vi "生成word报表.vi"(0 "Array输入":refnum<vi>, 1 "产品序号":string, 2 "标注图":T1(plugin-control), 3 "Array输入 2":refnum<vi>, 4 "测试人":string, 5 "部位":string, 6 "ROI左上角X":i32, 7 "ROI左上角Y":i32, 8 "反射图":T1(plugin-control) caption="Original Image", 9 "框号":dbl format="%#_13g") -> (14 "报告生成路径":path)   [LabVIEW 2018]
uses:
  <vilib>/Utility/NIReport.llb/Report Type.ctl
  <vilib>/Utility/NIReport.llb/Append Report Text (str wrap).vi
  <vilib>/addons/_office/word.llb/Word Edit Cell ([dbl]).vi
  <vilib>/addons/_office/word.llb/Word Edit Cell (str).vi
  <vilib>/Utility/NIReport.llb/Append Report Text (num wrap).vi
  <vilib>/Utility/NIReport.llb/NI_report.lvclass
  <vilib>/addons/_office/NI_ReportGenerationToolkit.lvlib
  <vilib>/Utility/NIReport.llb/Word/NI_Word.lvclass
  <vilib>/Utility/NIReport.llb/NI_ReportGenerationCore.lvlib
  <vilib>/addons/_office/word.llb/Word Edit Cell ([str]).vi
panel:
  out "绝对位置Y2":dbl[](array[numeric])
  out "绝对位置X2":dbl[](array[numeric])
  out "绝对位置Y":dbl[](array[numeric])
  out "绝对位置X":dbl[](array[numeric])
  out "分层累计缺陷占比":dbl
  out "分层Z值":dbl[](array[numeric])
  out "缺陷个数 2":i32
  out "分层数据":dbl[][](array[numeric])
  out "弥散累计缺陷占比":dbl
  out "弥散数据":dbl[][](array[numeric])
  out "弥散Z值":dbl[](array[numeric])
  out "缺陷个数":i32
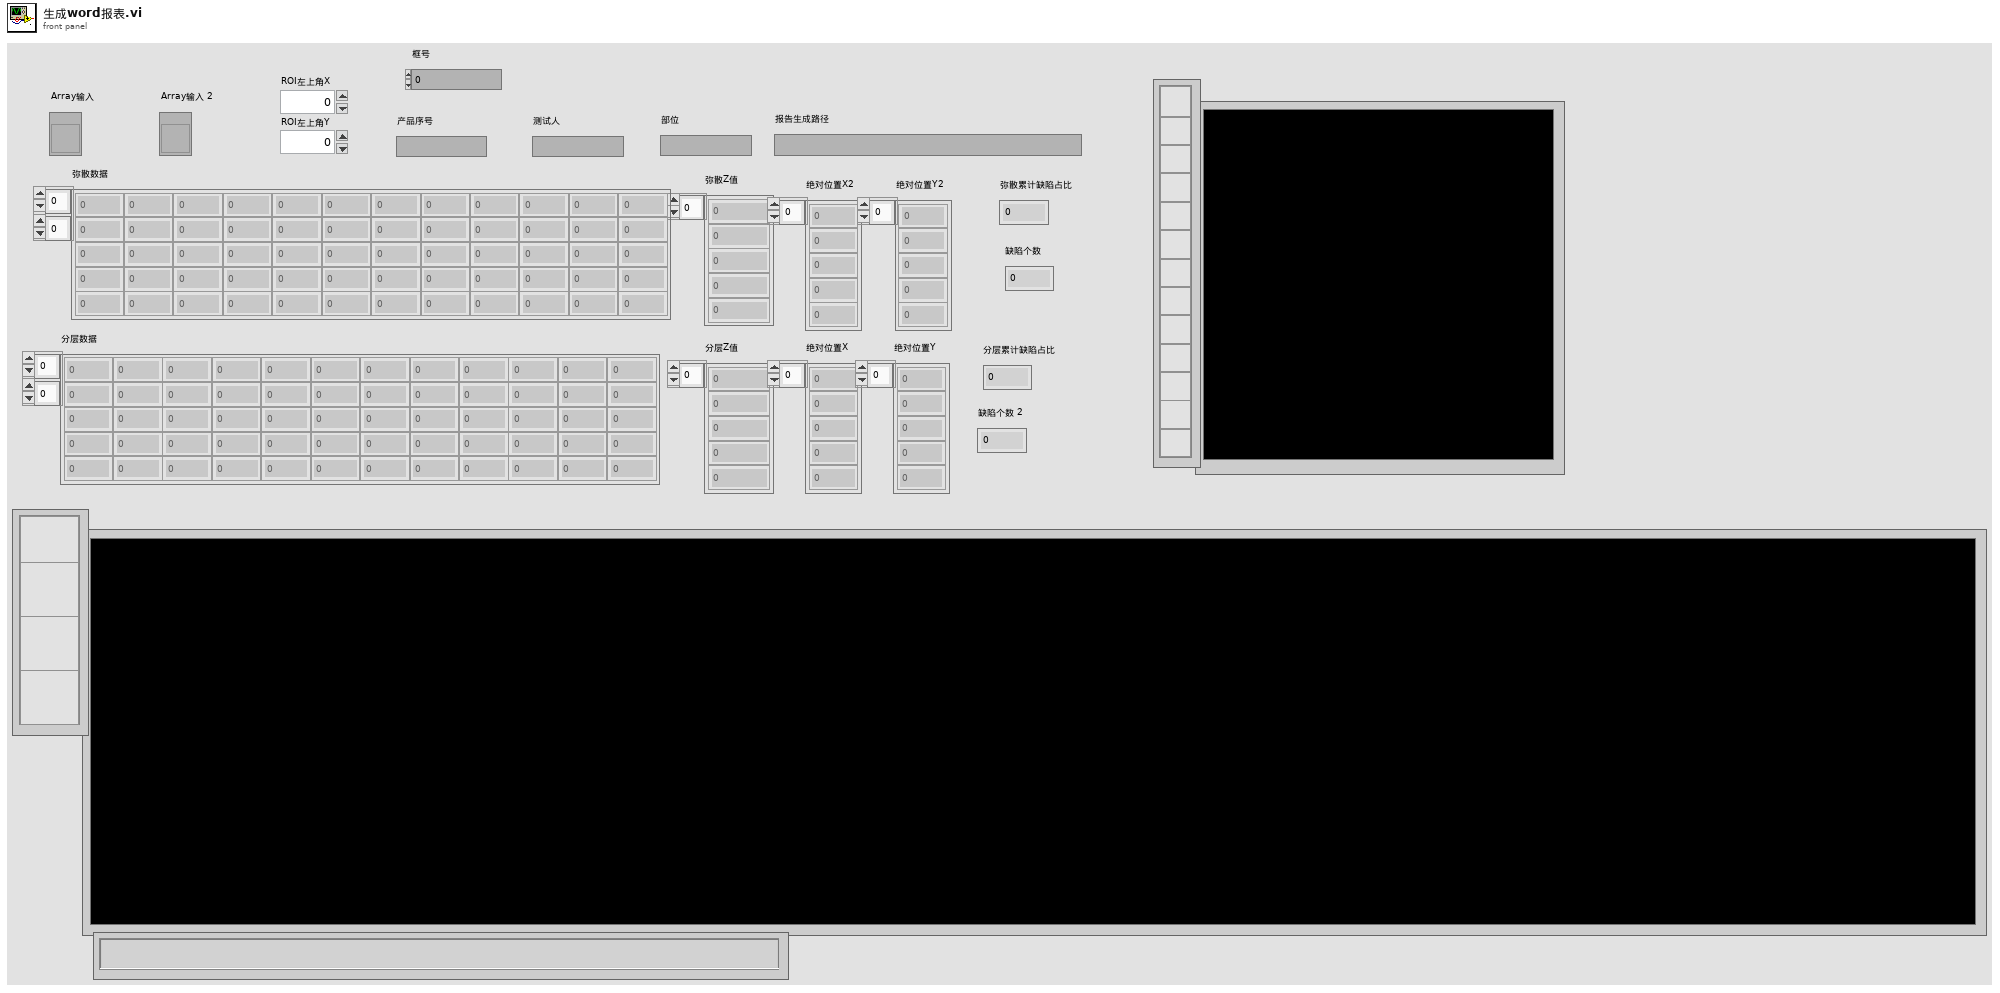
[diagram p1: front panel]
types:
  T1 = typedef "IMAQ Image.ctl" = refnum<image>
  T2 = cluster{"position (Excel)":cluster{"row":i32, "column":i32}, "name (Excel)":string, "bookmark (Word)":string}
  T3 = typedef "NI_ReportGenerationCore.lvlib/Report Type.ctl" = enum16{"HTML", "Word", "Excel"}
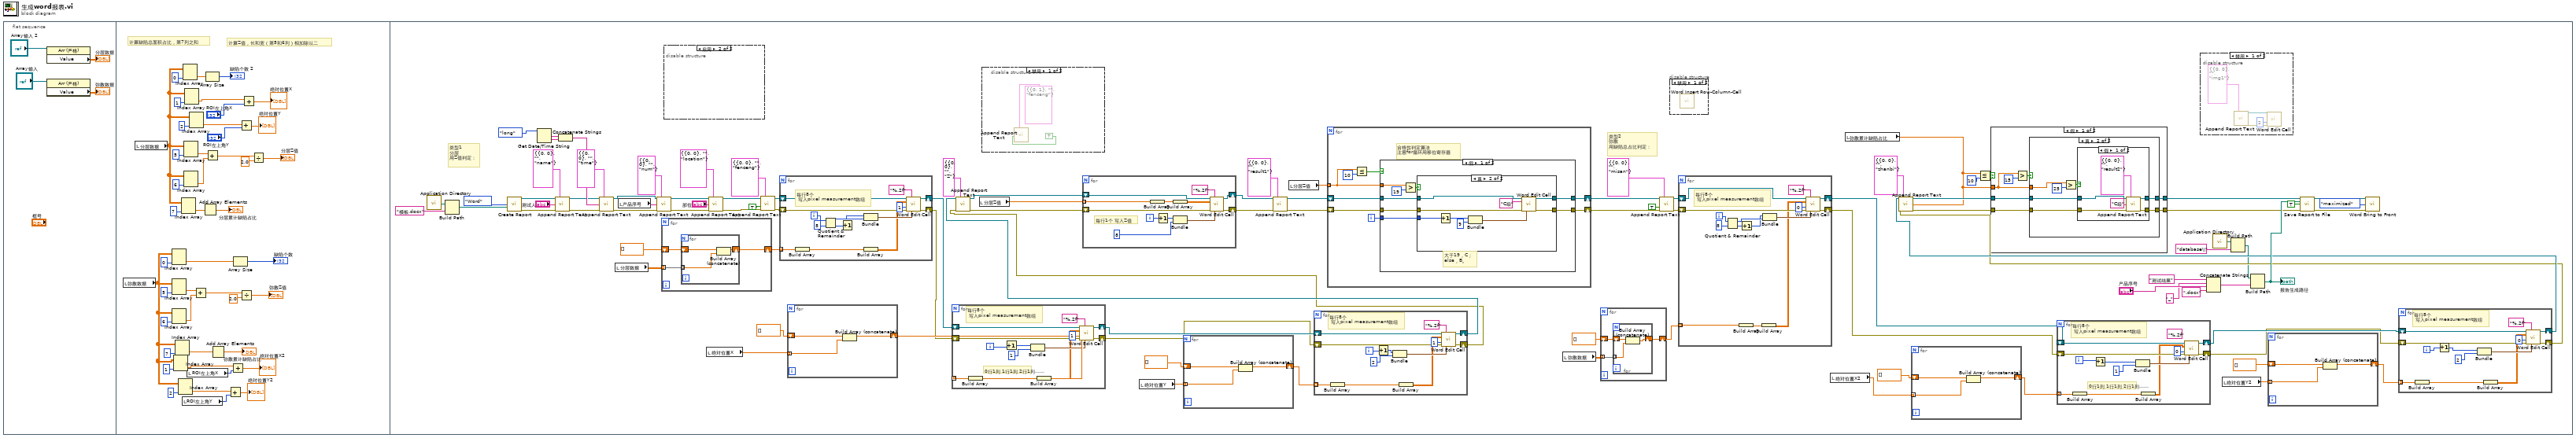
[diagram p0: block diagram]
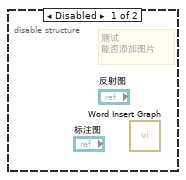
[diagram p5: hidden frame]
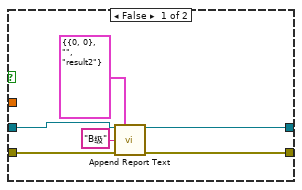
[diagram p6: hidden frame]
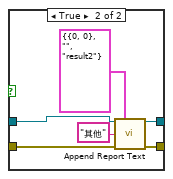
[diagram p7: hidden frame]
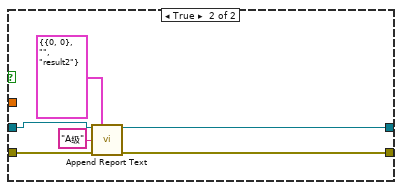
[diagram p8: hidden frame]
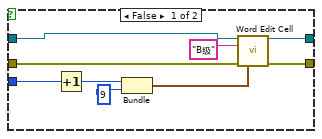
[diagram p9: hidden frame]
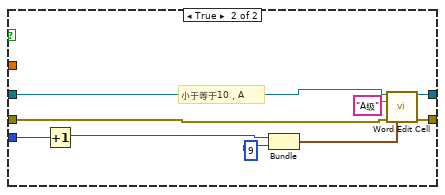
[diagram p10: hidden frame]
diagram:
  n1 = flat-sequence {
    frame #0 {
      n2 = property class="Arr (严格)"(reference="Array输入 2") -> ("Value"=→"分层数据":dbl[][])  [unwired: 1 in, 2 out]
      n3 = property class="Arr (严格)"(reference="Array输入") -> ("Value"=→"弥散数据":dbl[][])  [unwired: 1 in, 2 out]
    }
    frame #1 {
      # "计算缺陷总面积占比，第7列之和"
      # "计算Z值，长和宽（第5和6列）相加除以二"
      n4 = local read "弥散数据"() -> (w7:dbl[][])
      n5 = local read "分层数据"() -> (w20:dbl[][])
      n6 = Index Array(array=w7, index (col)=0 ("禁用的索引 (列)")) -> (element=w46:dbl[])  [unwired: 1 in]
      n7 = Index Array(array=w7, index (col)=5 ("索引")) -> (element=w43:dbl[])  [unwired: 1 in]
      n8 = Index Array(array=w7, index (col)=6 ("索引")) -> (element=w44:dbl[])  [unwired: 1 in]
      n9 = Index Array(array=w7, index (col)=1 ("索引 (列)")) -> (element=w11:dbl[])  [unwired: 1 in]
      n10 = Index Array(array=w7, index (col)=7 ("禁用的索引 (列)")) -> (element=w37:dbl[])  [unwired: 1 in]
      n11 = Index Array(array=w7, index (col)=2 ("索引 (列)")) -> (element=w9:dbl[])  [unwired: 1 in]
      n12 = Index Array(array=w20, index (col)=7 ("禁用的索引 (列)")) -> (element=w24:dbl[])  [unwired: 1 in]
      n13 = local read "ROI左上角Y"() -> (w5:i32)
      n14 = Index Array(array=w20, index (col)=0 ("禁用的索引 (列)")) -> (element=w33:dbl[])  [unwired: 1 in]
      n15 = Index Array(array=w20, index (col)=5 ("索引")) -> (element=w30:dbl[])  [unwired: 1 in]
      n16 = Index Array(array=w20, index (col)=6 ("索引")) -> (element=w31:dbl[])  [unwired: 1 in]
      n17 = Index Array(array=w20, index (col)=1 ("索引 (列)")) -> (element=w19:dbl[])  [unwired: 1 in]
      n18 = local read "ROI左上角X"() -> (w6:i32)
      n19 = Index Array(array=w20, index (col)=2 ("索引 (列)")) -> (element=w16:dbl[])  [unwired: 1 in]
      n20 = Add(x=w43, y=w44) -> (x+y=w45:dbl[])
      n21 = Add Array Elements(numeric array=w24) -> (sum=→"分层累计缺陷占比":dbl)
      n22 = Array Size(array=w33) -> (size(s)=→"缺陷个数 2":i32)
      n23 = Add(x=w30, y=w31) -> (x+y=w32:dbl[])
      n24 = Add Array Elements(numeric array=w37) -> (sum=→"弥散累计缺陷占比":dbl)
      n25 = Add(x=w9, y=w5) -> (x+y=→"绝对位置Y2":dbl[])
      n26 = Add(x=w11, y=w6) -> (x+y=→"绝对位置X2":dbl[])
      n27 = Array Size(array=w46) -> (size(s)=→"缺陷个数":i32)
      n28 = Add(x=w16, y="ROI左上角Y") -> (x+y=→"绝对位置Y":dbl[])
      n29 = Divide(x=w45, y=2.0) -> (x/y=→"弥散Z值":dbl[])
      n30 = Add(x=w19, y="ROI左上角X") -> (x+y=→"绝对位置X":dbl[])
      n31 = Divide(x=w32, y=2.0) -> (x/y=→"分层Z值":dbl[])
    }
    frame #2 {
      # "类型2\n弥散\n用缺陷总占比判定："
      # "类型1\n分层\n用Z值判定："
      n32 = call <vilib>:"Application Directory.vi"() -> ("Application Directory"=w128:path)
      n33 = Build Path(base path=w128, name or relative path="模板.docx") -> (appended path=w127:path)
      n34 = call <vilib>:"Create Report.vi"("report type"=Report_Type."Word" ("Report Type"), "template (empty)"=w127) -> ("report out"=w120:refnum<class "NI_report.lvclass">, "error out"=w117:errorcluster)  [unwired: 12 in]
      n35 = Get Date/Time String(date format (0)=enum16{"short", "long", "abbreviated"}."long" ("日期格式(0)")) -> (date string=w126:string, time string=w124:string)  [unwired: 2 in]
      n36 = call-poly <vilib>:"Append Report Text.vi"("report in"=w120, "MS Office parameters"=T2 {"position (Excel)"={"row"=0, "column"=0}, "name (Excel)"="", "bookmark (Word)"="name"}, "text"="测试人", "error in (no error)"=w117) -> ("report out"=w119:refnum<class "NI_report.lvclass">, "error out"=w118:errorcluster)  [unwired: 8 in, 2 out]
      n37 = Concatenate Strings(w126, w124) -> (w125:string)
      n38 = call-poly <vilib>:"Append Report Text.vi"("report in"=w119, "MS Office parameters"=T2 {"position (Excel)"={"row"=0, "column"=0}, "name (Excel)"="", "bookmark (Word)"="time"}, "text"=w125, "error in (no error)"=w118) -> ("report out"=w123:refnum<class "NI_report.lvclass">, "error out"=w122:errorcluster)  [unwired: 8 in, 2 out]
      n39 = local read "分层数据"() -> (w131:dbl[][])
      n40 = local read "产品序号"() -> (w95:string)
      n41 = call-poly <vilib>:"Append Report Text.vi"("report in"=w123, "MS Office parameters"=T2 {"position (Excel)"={"row"=0, "column"=0}, "name (Excel)"="", "bookmark (Word)"="num"}, "text"=w95, "error in (no error)"=w122) -> ("report out"=w97:refnum<class "NI_report.lvclass">, "error out"=w96:errorcluster)  [unwired: 8 in, 2 out]
      n42 = for {
        tunnel: w131 -> [w330] mode=indexing
        shift-right: [w328] -> w121
        shift-left: dbl[] [] ("元素") -> [w329]
        n43 = for {
          tunnel: w330 -> [w333] mode=indexing
          shift-right: [w331] -> w328
          shift-left: w329 -> [w332]
          n44 = Build Array (concatenate)(w332, w333) -> (w331:dbl[])
        }
      }
      n45 = disable-structure shown="启用" {
        frame Disabled {
          # "测试\n能否添加图片"
          n46 = call <vilib>:"Word Insert Graph.vi"() -> ()  [unwired: 12 in, 4 out]
        }
        frame Enabled {
        }
      }
      n47 = local read "绝对位置X"() -> (w75:dbl[])
      n48 = call-poly <vilib>:"Append Report Text.vi"("report in"=w97, "MS Office parameters"=T2 {"position (Excel)"={"row"=0, "column"=0}, "name (Excel)"="", "bookmark (Word)"="location"}, "text"="部位", "error in (no error)"=w96) -> ("report out"=w99:refnum<class "NI_report.lvclass">, "error out"=w98:errorcluster)  [unwired: 8 in, 2 out]
      n49 = call-poly <vilib>:"Append Report Text.vi"("report in"=w99, "MS Office parameters"=T2 {"position (Excel)"={"row"=0, "column"=0}, "name (Excel)"="", "bookmark (Word)"="fenceng"}, "append on new line? (F)"=TRUE, "error in (no error)"=w98) -> ("report out"=w130:refnum<class "NI_report.lvclass">, "error out"=w129:errorcluster)  [unwired: 8 in, 2 out]
      n50 = for {
        shift-right: [w348] -> w55
        shift-left: w130 -> [w343]
        shift-right: [w347] -> w54
        shift-left: w129 -> [w342]
        tunnel: w121 -> [w336] mode=indexing
        i -> [w344]
        # "每行8个\n 写入pixel measurement数组"
        n51 = Build Array(w336) -> (w338:dbl[])
        n52 = Quotient & Remainder(x=w344, y=8) -> (x-y*floor(x/y)=w341:i32, floor(x/y)=w340:i32)
        n53 = Increment(x=w340) -> (x+1=w339:i32)
        n54 = Bundle(w339, w341) -> (w346:cluster{i32, i32})  [unwired: 1 in]
        n55 = Build Array(w338) -> (w337:dbl[][])
        n56 = call-poly <vilib>:"Word Edit Cell.vi"("report in"=w343, "format string (%.3f)"="%.2f", "value"=w337, "table index (-1)"=i16 1, "error in (no error)"=w342, "start (0, 0)"=w346) -> ("report out"=w348:refnum<class "NI_report.lvclass">, "error out"=w347:errorcluster)  [unwired: 8 in]
      }
      n57 = for {
        tunnel: w75 -> [w196] mode=indexing
        shift-right: [w194] -> w74
        shift-left: dbl[] [] ("元素") -> [w195]
        n58 = Build Array (concatenate)(w195, w196) -> (w194:dbl[])
      }
      n59 = for {
        shift-right: [w209] -> w71
        shift-left: w55 -> [w206]
        shift-right: [w208] -> w70
        shift-left: w54 -> [w205]
        tunnel: w74 -> [w202] mode=indexing
        i -> [w198]
        # "0行1列 1行1列 2行1列......"
        # "每行8个\n 写入pixel measurement数组"
        n60 = Build Array(w202) -> (w204:dbl[])
        n61 = Increment(x=w198) -> (x+1=w197:i32)
        n62 = Bundle(w197, 1) -> (w207:cluster{i32, i32})  [unwired: 1 in]
        n63 = Build Array(w204) -> (w203:dbl[][])
        n64 = call-poly <vilib>:"Word Edit Cell.vi"("report in"=w206, "format string (%.3f)"="%.2f", "value"=w203, "table index (-1)"=i16 1, "error in (no error)"=w205, "start (0, 0)"=w207) -> ("report out"=w209:refnum<class "NI_report.lvclass">, "error out"=w208:errorcluster)  [unwired: 8 in]
      }
      n65 = local read "分层Z值"() -> (w132:dbl[])
      n66 = disable-structure shown="禁用" {
        frame Disabled {
          n67 = call-poly <vilib>:"Append Report Text.vi"("MS Office parameters"=T2 {"position (Excel)"={"row"=0, "column"=1}, "name (Excel)"="", "bookmark (Word)"="fenceng"}, "append on new line? (F)"=TRUE) -> ()  [unwired: 10 in, 4 out]
        }
        frame Enabled {
        }
      }
      n68 = local read "绝对位置Y"() -> (w73:dbl[])
      n69 = for {
        tunnel: w73 -> [w180] mode=indexing
        shift-right: [w178] -> w72
        shift-left: dbl[] [] ("元素") -> [w179]
        n70 = Build Array (concatenate)(w179, w180) -> (w178:dbl[])
      }
      n71 = local read "分层Z值"() -> (w133:dbl[])
      n72 = for {
        shift-right: [w193] -> w69
        shift-left: w71 -> [w190]
        shift-right: [w192] -> w68
        shift-left: w70 -> [w189]
        tunnel: w72 -> [w186] mode=indexing
        i -> [w182]
        # "每行8个\n 写入pixel measurement数组"
        n73 = Build Array(w186) -> (w188:dbl[])
        n74 = Increment(x=w182) -> (x+1=w181:i32)
        n75 = Bundle(w181, 2) -> (w191:cluster{i32, i32})  [unwired: 1 in]
        n76 = Build Array(w188) -> (w187:dbl[][])
        n77 = call-poly <vilib>:"Word Edit Cell.vi"("report in"=w190, "format string (%.3f)"="%.2f", "value"=w187, "table index (-1)"=i16 1, "error in (no error)"=w189, "start (0, 0)"=w191) -> ("report out"=w193:refnum<class "NI_report.lvclass">, "error out"=w192:errorcluster)  [unwired: 8 in]
      }
      n78 = call-poly <vilib>:"Append Report Text.vi"("report in"=w69, "MS Office parameters"=T2 {"position (Excel)"={"row"=0, "column"=0}, "name (Excel)"="", "bookmark (Word)"="Z"}, "error in (no error)"=w68) -> ("report out"=w139:refnum<class "NI_report.lvclass">, "error out"=w138:errorcluster)  [unwired: 9 in, 2 out]
      n79 = for {
        shift-right: [w327] -> w135
        shift-left: w139 -> [w324]
        shift-right: [w326] -> w134
        shift-left: w138 -> [w323]
        tunnel: w132 -> [w319] mode=indexing
        i -> [w317]
        # "每行1个 写入Z值"
        n80 = Build Array(w319) -> (w321:dbl[])
        n81 = Increment(x=w317) -> (x+1=w322:i32)
        n82 = Build Array(w321) -> (w320:dbl[][])
        n83 = Bundle(w322, "y"=8) -> (w325:cluster{i32, "y":i32})  [unwired: 1 in]
        n84 = call-poly <vilib>:"Word Edit Cell.vi"("report in"=w324, "format string (%.3f)"="%.2f", "value"=w320, "error in (no error)"=w323, "start (0, 0)"=w325) -> ("report out"=w327:refnum<class "NI_report.lvclass">, "error out"=w326:errorcluster)  [unwired: 9 in]
      }
      n85 = call-poly <vilib>:"Append Report Text.vi"("report in"=w135, "MS Office parameters"=T2 {"position (Excel)"={"row"=0, "column"=0}, "name (Excel)"="", "bookmark (Word)"="result1"}, "error in (no error)"=w134) -> ("report out"=w136:refnum<class "NI_report.lvclass">, "error out"=w137:errorcluster)  [unwired: 9 in, 2 out]
      n86 = for {
        shift-right: [w274] -> w92
        shift-left: w136 -> [w277]
        shift-right: [w275] -> w91
        shift-left: w137 -> [w276]
        tunnel: w133 -> [w273] mode=indexing
        i -> [w278]
        # "合格性判定算法\n注意for循环用移位寄存器"
        n87 = Less Or Equal?(x=w273, y=10) -> (x <= y?=w279:bool)
        n88 = case shown="假" w279 {
          tunnel: w278 -> [w285 w313]
          tunnel: w277 -> [w284 w312]
          tunnel: w276 -> [w283 w311]
          tunnel: [w281 w310] -> w275
          tunnel: [w282 w309] -> w274
          tunnel: w273 -> [w288 _]
          frame False {
            # "大于19，C；\nelse，B。"
            n89 = Greater?(x=w288, y=19) -> (0:w286:bool)
            n90 = case shown="真" w286 {
              tunnel: w285 -> [w289 w302]
              tunnel: w284 -> [w293 w301]
              tunnel: w283 -> [w292 w300]
              tunnel: [w291 w299] -> w282
              tunnel: [w290 w298] -> w281
              frame False {
                n91 = Increment(x=w289) -> (x+1=w297:i32)
                n92 = Bundle(w297, "y"=9) -> (w296:cluster{i32, "y":i32})  [unwired: 1 in]
                n93 = call-poly <vilib>:"Word Edit Cell.vi"("report in"=w293, "value"="B级", "error in (no error)"=w292, "start (0, 0)"=w296) -> ("report out"=w291:refnum<class "NI_report.lvclass">, "error out"=w290:errorcluster)  [unwired: 10 in]
              }
              frame True {
                n94 = Increment(x=w302) -> (x+1=w306:i32)
                n95 = Bundle(w306, "y"=9) -> (w305:cluster{i32, "y":i32})  [unwired: 1 in]
                n96 = call-poly <vilib>:"Word Edit Cell.vi"("report in"=w301, "value"="C级", "error in (no error)"=w300, "start (0, 0)"=w305) -> ("report out"=w299:refnum<class "NI_report.lvclass">, "error out"=w298:errorcluster)  [unwired: 10 in]
              }
            }
          }
          frame True {
            # "小于等于10，A"
            n97 = Increment(x=w313) -> (x+1=w315:i32)
            n98 = Bundle(w315, "y"=9) -> (w307:cluster{i32, "y":i32})  [unwired: 1 in]
            n99 = call-poly <vilib>:"Word Edit Cell.vi"("report in"=w312, "value"="A级", "error in (no error)"=w311, "start (0, 0)"=w307) -> ("report out"=w309:refnum<class "NI_report.lvclass">, "error out"=w310:errorcluster)  [unwired: 10 in]
          }
        }
      }
      n100 = local read "弥散数据"() -> (w90:dbl[][])
      n101 = for {
        tunnel: w90 -> [w269] mode=indexing
        shift-right: [w267] -> w86
        shift-left: dbl[] [] ("元素") -> [w268]
        n102 = for {
          tunnel: w269 -> [w272] mode=indexing
          shift-right: [w270] -> w267
          shift-left: w268 -> [w271]
          n103 = Build Array (concatenate)(w271, w272) -> (w270:dbl[])
        }
      }
      n104 = call-poly <vilib>:"Append Report Text.vi"("report in"=w92, "MS Office parameters"=T2 {"position (Excel)"={"row"=0, "column"=0}, "name (Excel)"="", "bookmark (Word)"="misan"}, "append on new line? (F)"=TRUE, "error in (no error)"=w91) -> ("report out"=w88:refnum<class "NI_report.lvclass">, "error out"=w87:errorcluster)  [unwired: 8 in, 2 out]
      n105 = disable-structure shown="禁用" {
        frame Disabled {
          n106 = call <vilib>:"Word Insert Row-Column-Cell.vi"() -> ()  [unwired: 14 in, 2 out]
        }
        frame Enabled {
        }
      }
      n107 = for {
        shift-right: [w266] -> w53
        shift-left: w88 -> [w261]
        shift-right: [w265] -> w52
        shift-left: w87 -> [w260]
        tunnel: w86 -> [w254] mode=indexing
        i -> [w262]
        # "每行8个\n 写入pixel measurement数组"
        n108 = Quotient & Remainder(x=w262, y=8) -> (x-y*floor(x/y)=w259:i32, floor(x/y)=w258:i32)
        n109 = Build Array(w254) -> (w256:dbl[])
        n110 = Increment(x=w258) -> (x+1=w257:i32)
        n111 = Build Array(w256) -> (w255:dbl[][])
        n112 = Bundle(w257, w259) -> (w264:cluster{i32, i32})  [unwired: 1 in]
        n113 = call-poly <vilib>:"Word Edit Cell.vi"("report in"=w261, "format string (%.3f)"="%.2f", "value"=w255, "table index (-1)"=i16 0, "error in (no error)"=w260, "start (0, 0)"=w264) -> ("report out"=w266:refnum<class "NI_report.lvclass">, "error out"=w265:errorcluster)  [unwired: 8 in]
      }
      n114 = local read "绝对位置X2"() -> (w57:dbl[])
      n115 = local read "弥散累计缺陷占比"() -> (w80:dbl)
      n116 = for {
        tunnel: w57 -> [w177] mode=indexing
        shift-right: [w175] -> w67
        shift-left: dbl[] [] ("元素") -> [w176]
        n117 = Build Array (concatenate)(w176, w177) -> (w175:dbl[])
      }
      n118 = Less Or Equal?(x=w80, y=10) -> (x <= y?=w81:bool)
      n119 = for {
        shift-right: [w174] -> w64
        shift-left: w53 -> [w171]
        shift-right: [w173] -> w63
        shift-left: w52 -> [w170]
        tunnel: w67 -> [w167] mode=indexing
        i -> [w164]
        (unwired) "%.2f" ("format string (%.3f)")
        # "0行1列 1行1列 2行1列......"
        # "每行8个\n 写入pixel measurement数组"
        n120 = Build Array(w167) -> (w166:dbl[])
        n121 = Increment(x=w164) -> (x+1=w163:i32)
        n122 = Bundle(w163, 1) -> (w172:cluster{i32, i32})  [unwired: 1 in]
        n123 = Build Array(w166) -> (w165:dbl[][])
        n124 = call-poly <vilib>:"Word Edit Cell.vi"("report in"=w171, "value"=w165, "table index (-1)"=i16 0, "error in (no error)"=w170, "start (0, 0)"=w172) -> ("report out"=w174:refnum<class "NI_report.lvclass">, "error out"=w173:errorcluster)  [unwired: 9 in]
      }
      n125 = disable-structure shown="禁用" {
        frame Disabled {
          n126 = call-poly <vilib>:"Append Report Text.vi"("MS Office parameters"=T2 {"position (Excel)"={"row"=0, "column"=0}, "name (Excel)"="", "bookmark (Word)"="img1"}) -> ("report out"=w212:refnum<class "NI_report.lvclass">, "error out"=w211:errorcluster)  [unwired: 11 in, 2 out]
          n127 = call-poly <vilib>:"Word Edit Cell.vi"("report in"=w212, "table index (-1)"=i16 2, "error in (no error)"=w211) -> ()  [unwired: 11 in, 2 out]
        }
        frame Enabled {
        }
      }
      n128 = Concatenate Strings("测试结果" ("字符串"), "_" ("名称或相对路径"), "产品序号", ".docx" ("名称或相对路径")) -> (w143:string)
      n129 = call <vilib>:"Application Directory.vi"() -> ("Application Directory"=w51:path)
      n130 = local read "绝对位置Y2"() -> (w65:dbl[])
      n131 = Build Path(base path=w51, name or relative path="database\\" ("名称或相对路径")) -> (appended path=w49:path)
      n132 = Build Path(base path=w49, name or relative path=w143) -> (appended path=w144:path)
      "报告生成路径" <- w144
      n133 = for {
        tunnel: w65 -> [w149] mode=indexing
        shift-right: [w147] -> w66
        shift-left: dbl[] [] ("元素") -> [w148]
        n134 = Build Array (concatenate)(w148, w149) -> (w147:dbl[])
      }
      n135 = for {
        shift-right: [w162] -> w62
        shift-left: w64 -> [w159]
        shift-right: [w161] -> w61
        shift-left: w63 -> [w158]
        tunnel: w66 -> [w155] mode=indexing
        i -> [w151]
        # "每行8个\n 写入pixel measurement数组"
        n136 = Build Array(w155) -> (w157:dbl[])
        n137 = Increment(x=w151) -> (x+1=w150:i32)
        n138 = Bundle(w150, 2) -> (w160:cluster{i32, i32})  [unwired: 1 in]
        n139 = Build Array(w157) -> (w156:dbl[][])
        n140 = call-poly <vilib>:"Word Edit Cell.vi"("report in"=w159, "format string (%.3f)"="%.2f", "value"=w156, "table index (-1)"=i16 0, "error in (no error)"=w158, "start (0, 0)"=w160) -> ("report out"=w162:refnum<class "NI_report.lvclass">, "error out"=w161:errorcluster)  [unwired: 8 in]
      }
      n141 = call-poly <vilib>:"Append Report Text.vi"("report in"=w62, "MS Office parameters"=T2 {"position (Excel)"={"row"=0, "column"=0}, "name (Excel)"="", "bookmark (Word)"="zhanbi"}, "text"=w80, "error in (no error)"=w61) -> ("report out"=w84:refnum<class "NI_report.lvclass">, "error out"=w83:errorcluster)  [unwired: 8 in, 2 out]
      n142 = case shown="假" w81 {
        tunnel: w84 -> [w218 w249]
        tunnel: w83 -> [w216 w248]
        tunnel: [w215 w247] -> w76
        tunnel: [w217 w246] -> w77
        tunnel: w80 -> [w214 _]
        frame False {
          n143 = Greater?(x=w214, y=15) -> (0:w219:bool)
          n144 = case shown="真" w219 {
            tunnel: w218 -> [w224 w230]
            tunnel: [w223 w227] -> w217
            tunnel: w216 -> [w222 w229]
            tunnel: [w221 w228] -> w215
            tunnel: w214 -> [_ w232]
            frame False {
              n145 = call-poly <vilib>:"Append Report Text.vi"("report in"=w224, "MS Office parameters"=T2 {"position (Excel)"={"row"=0, "column"=0}, "name (Excel)"="", "bookmark (Word)"="result2"}, "text"="B级", "error in (no error)"=w222) -> ("report out"=w223:refnum<class "NI_report.lvclass">, "error out"=w221:errorcluster)  [unwired: 8 in, 2 out]
            }
            frame True {
              n146 = Greater?(x=w232, y=25) -> (0:w231:bool)
              n147 = case shown="假" w231 {
                tunnel: w230 -> [w237 w243]
                tunnel: w229 -> [w236 w242]
                tunnel: [w235 w241] -> w228
                tunnel: [w234 w240] -> w227
                frame False {
                  n148 = call-poly <vilib>:"Append Report Text.vi"("report in"=w237, "MS Office parameters"=T2 {"position (Excel)"={"row"=0, "column"=0}, "name (Excel)"="", "bookmark (Word)"="result2"}, "text"="C级", "error in (no error)"=w236) -> ("report out"=w234:refnum<class "NI_report.lvclass">, "error out"=w235:errorcluster)  [unwired: 8 in, 2 out]
                }
                frame True {
                  n149 = call-poly <vilib>:"Append Report Text.vi"("report in"=w243, "MS Office parameters"=T2 {"position (Excel)"={"row"=0, "column"=0}, "name (Excel)"="", "bookmark (Word)"="result2"}, "text"="其他", "error in (no error)"=w242) -> ("report out"=w240:refnum<class "NI_report.lvclass">, "error out"=w241:errorcluster)  [unwired: 8 in, 2 out]
                }
              }
            }
          }
        }
        frame True {
          n150 = call-poly <vilib>:"Append Report Text.vi"("report in"=w249, "MS Office parameters"=T2 {"position (Excel)"={"row"=0, "column"=0}, "name (Excel)"="", "bookmark (Word)"="result2"}, "text"="A级", "error in (no error)"=w248) -> ("report out"=w246:refnum<class "NI_report.lvclass">, "error out"=w247:errorcluster)  [unwired: 8 in, 2 out]
        }
      }
      n151 = call-dynamic "Save Report to File.vi"("report in"=w77, "report file path"=w144, "prompt to replace? (F)"=TRUE, "error in (no error)"=w76) -> ("report out"=w142:refnum<class "NI_report.lvclass">, "error out"=w141:errorcluster)  [unwired: 10 in]
      n152 = call <vilib>:"Word Bring to Front.vi"("report in"=w142, "window state (maximized)"=enum16{"maximized", "minimized", "normal"}."maximized", "error in (no error)"=w141) -> ()  [unwired: 11 in, 2 out]
    }
  }
